vi "Merge Array Elements at Path.vi"(8 "error in (no error)":errorcluster, 9 "Slot Topology Variant":variant, 10 "Path String":string, 11 "Base Topology Variant":variant) -> (0 "error out":errorcluster, 3 "Base Topology Variant out":variant)   [LabVIEW 2017]
uses:
  <vilib>/National Instruments/Variant Data Manipulation/Path API/Read Value at Path(String).vi
  <vilib>/National Instruments/Variant Data Manipulation/Path API/Write Value at Path(String).vi
  <vilib>/National Instruments/Variant Data Manipulation/Variant Data Manipulation.lvlib
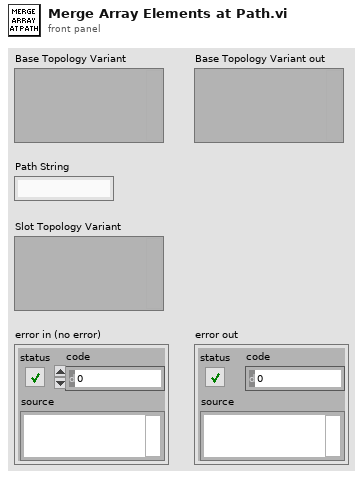
[diagram p1: front panel]
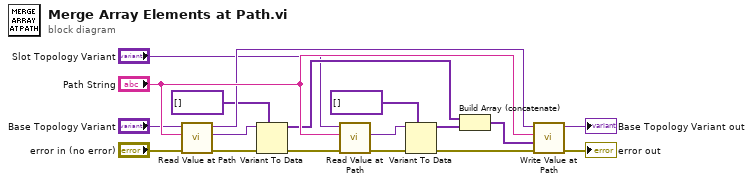
[diagram p0: block diagram]
diagram:
  n1 = call-poly <vilib>:"Read Value at Path.vi"("error in (no error)"="error in (no error)", "Path String"="Path String", "Variant in"="Base Topology Variant") -> ("error out"=w11:errorcluster, "Element out"=w6:variant, "Variant out"=w15:variant)  [unwired: 6 in]
  n2 = Variant To Data(error in=w11, type=variant[] [], Variant=w6) -> (data=w13:variant[], error out=w3:errorcluster)
  n3 = call-poly <vilib>:"Read Value at Path.vi"("error in (no error)"=w3, "Path String"="Path String", "Variant in"="Slot Topology Variant") -> ("error out"=w12:errorcluster, "Element out"=w9:variant)  [unwired: 6 in, 1 out]
  n4 = Variant To Data(error in=w12, type=variant[] [], Variant=w9) -> (data=w14:variant[], error out=w2:errorcluster)
  n5 = Build Array (concatenate)(w13, w14) -> (w17:variant[])
  n6 = call-poly <vilib>:"Write Value at Path.vi"("error in (no error)"=w2, "Element in"=w17, "Path String"="Path String", "Variant in"=w15) -> ("error out"=→"error out":errorcluster, "Variant out"=→"Base Topology Variant out":variant)  [unwired: 6 in]
